vi "READ_ADC_Command.vi"(9 "Canal":u8, 10 "Marca":T1) -> (1 "length":i32, 2 "Expected Response":string, 3 "Command":string, 4 "Bytes Expected":u32=2)   [LabVIEW 2019, in "Serial Device.lvclass"]
uses:
  Serial Device.lvclass
  Marca.ctl
  Comando.ctl
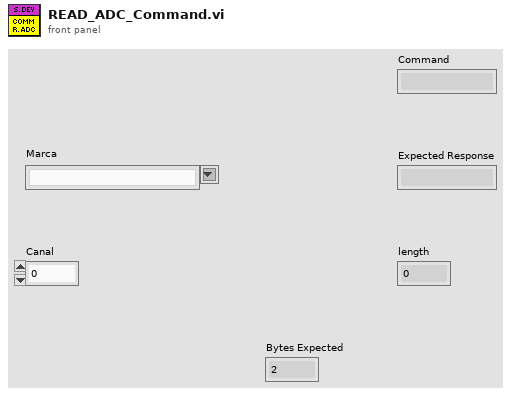
[diagram p1: front panel]
types:
  T1 = typedef "Marca.ctl" = string
  T2 = typedef "Comando.ctl" = string
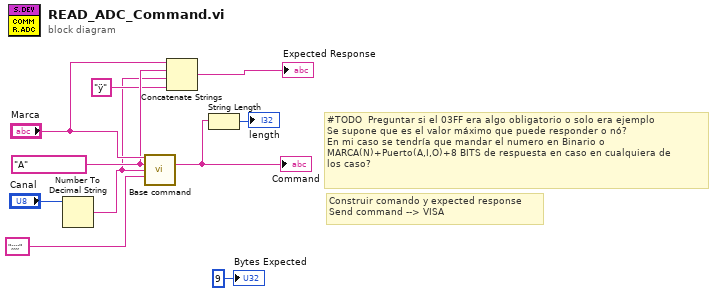
[diagram p0: block diagram]
diagram:
  w8 = T2 "A" ("Comando")
  # "Construir comando y expected response\nSend command --> VISA"
  # "#TODO  Preguntar si el 03FF era algo obligatorio o solo era ejemplo\nSe supone que es el valor máximo que puede responder o nó?\nEn mi caso se tendría que mandar el numero en Binario o \nMARCA(N)+Puerto(A,I,O)+8 BITS de respuesta en caso en cualquiera de \nlos caso?"
  n1 = Number To Decimal String(number="Canal") -> (decimal integer string=w1:string)  [unwired: 1 in]
  n2 = call "Base command.vi"("Marca"="Marca", "Comando"=w8, "Parametro 1"=w1, "Parametro 2"=";;;;") -> ("Command"=w6:string)  [unwired: 10 in, 1 out]
  "Command" <- w6
  n3 = Concatenate Strings("Marca", w8, w1, "ÿ") -> (→"Expected Response":string)
  n4 = String Length(string=w6) -> (length=→"length":i32)
  "Bytes Expected" <- u32 9 ("byte count")
